vi "model torque calculation3MathScript.vi"() -> ()   [LabVIEW 2019]
uses:
  <vilib>/imath/engines/lvmath2/RunTimeEngine/NodeEndStatement/NIMS_NodeEndStatement_Output.vi
  <instcachedir>/0/NIMS_NodeEndStatement_Output_53EC0D466D134D7ABD903AC30B43404B.lvgen/NIMS_NodeEndStatement_Output_53EC0D466D134D7ABD903AC30B43404B_001.vi
  <vilib>/imath/engines/lvmath2/RunTimeEngine/ErrorHandling/NIMS_Finalize Error.vi
panel:
  out "lower leg(l2)":dbl(slide) scale=8.0..48.0
  out "foot(l3)":dbl(slide) scale=2.0..12.0
  out "thigh(l1)":dbl(slide) scale=8.0..48.0
  out "Tknee":dbl(slide) scale=-100.0..200.0
  out "Tankle":dbl(slide) scale=-100.0..200.0
  out "Thip":dbl(slide) scale=-100.0..200.0
  in  "?":dbl(slide) scale=40.0..190.0
  in  "Ankle_è3":dbl(slide) scale=-45.0..45.0
  in  "Knee_è2":dbl(slide) scale=0.0..145.0
  in  "hip_è1":dbl(slide) scale=-10.0..145.0
  in  "Select Model BSP":bool
  in  "Select sex":bool
  out "KneeD_m4":dbl(slide) scale=0.0..35.0
  out "FootD_m3":dbl(slide) scale=0.0..4.0
  out "LowerLegD_m2":dbl(slide) scale=0.0..10.0
  out "ThighD_m1":dbl(slide) scale=0.0..25.0 scale format="%#.8g"
  in  "?":dbl(slide) scale=20.0..170.0
  # "CALCULATION OF BASIC SIZES OF ROBOTIC EXTRACTUAL LOWER LIMB"
  # "KINEMATIC ANALYSIS"
  # "Á.Calculate the mass of each member of the lower limb in relation to its total mass"
  # "Mass Segment Body to Model Dempster BSP"
  # "Select Total Mass(Kg)"
  # "Zatsiorsky BSP"
  # "Dempster BSP"
  # "Males"
  # "Female"
  # "B.Calculation of moments of each segment  of the lower right extremity in relation to the total mass (kg) its height (m) and the change of angles of each joints."
  # "Select Angles"
  # "Select Height(h)"
  # "Length(cm)"
  # "Flexion/extension"
  # "m"
  # "Nm"
  # "Nm"
  # "Nm"
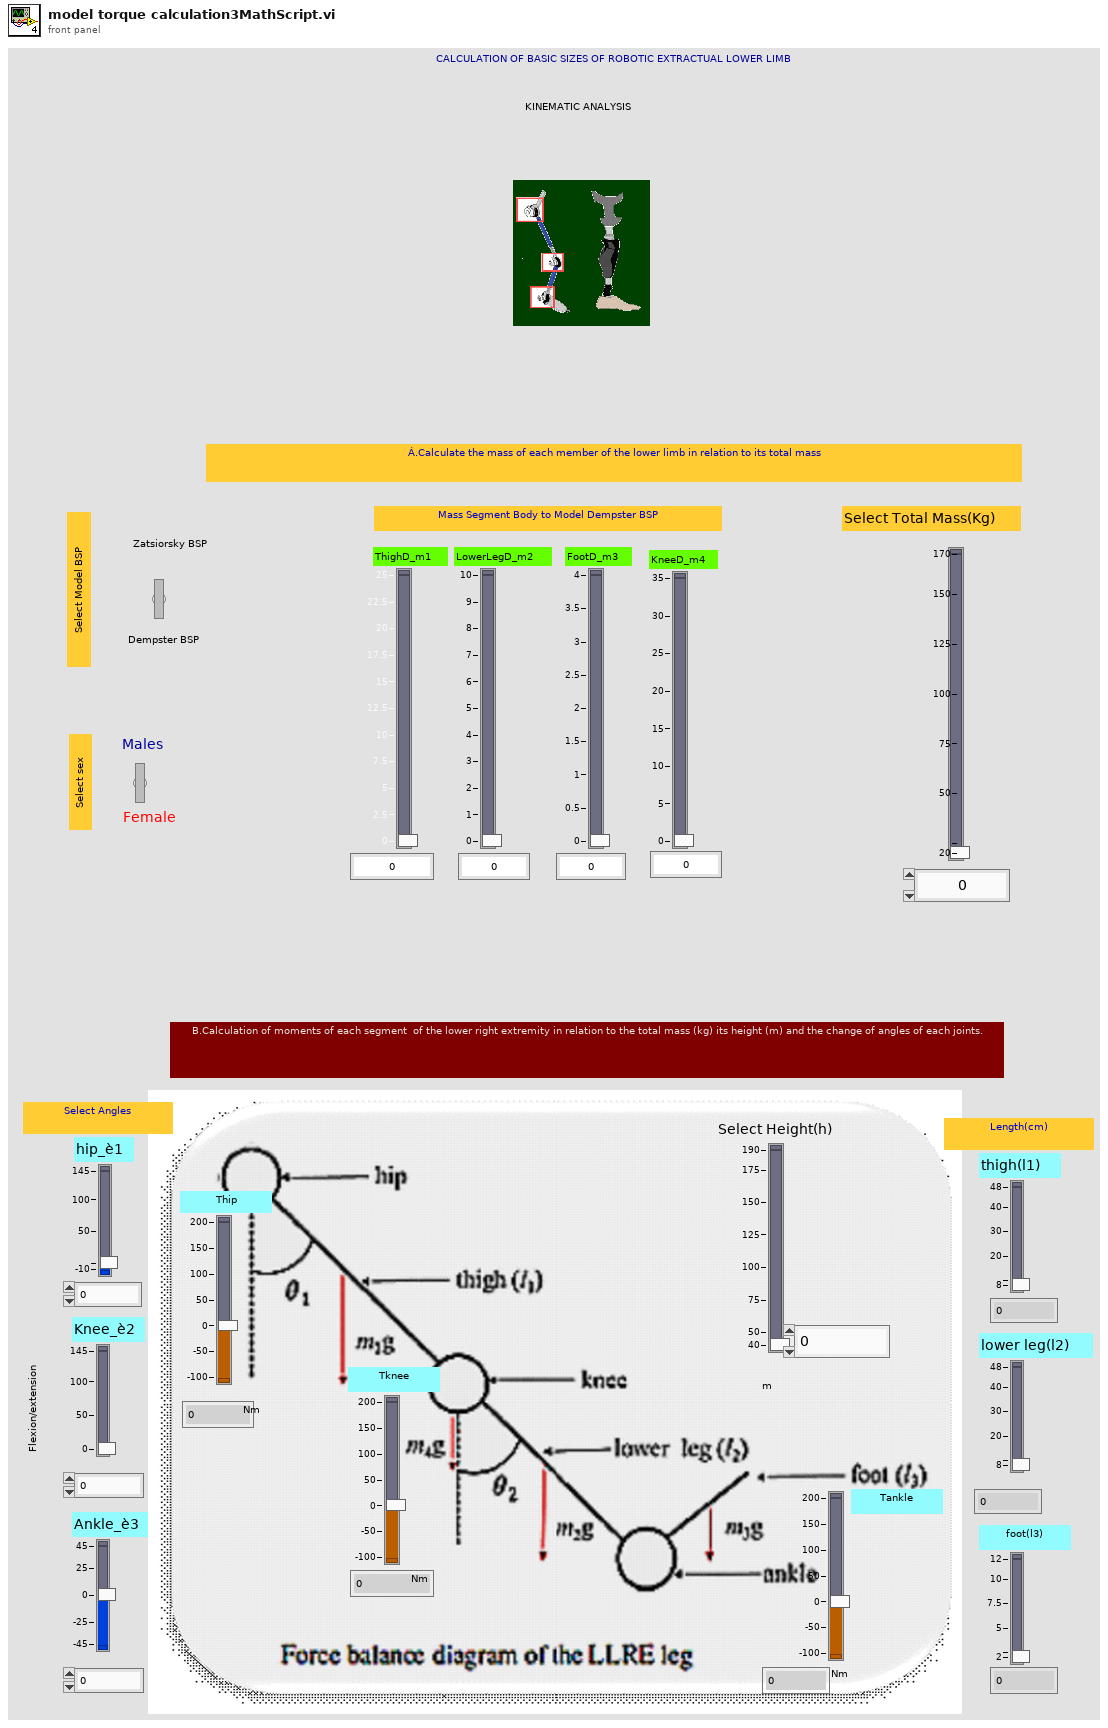
[diagram p1: front panel]
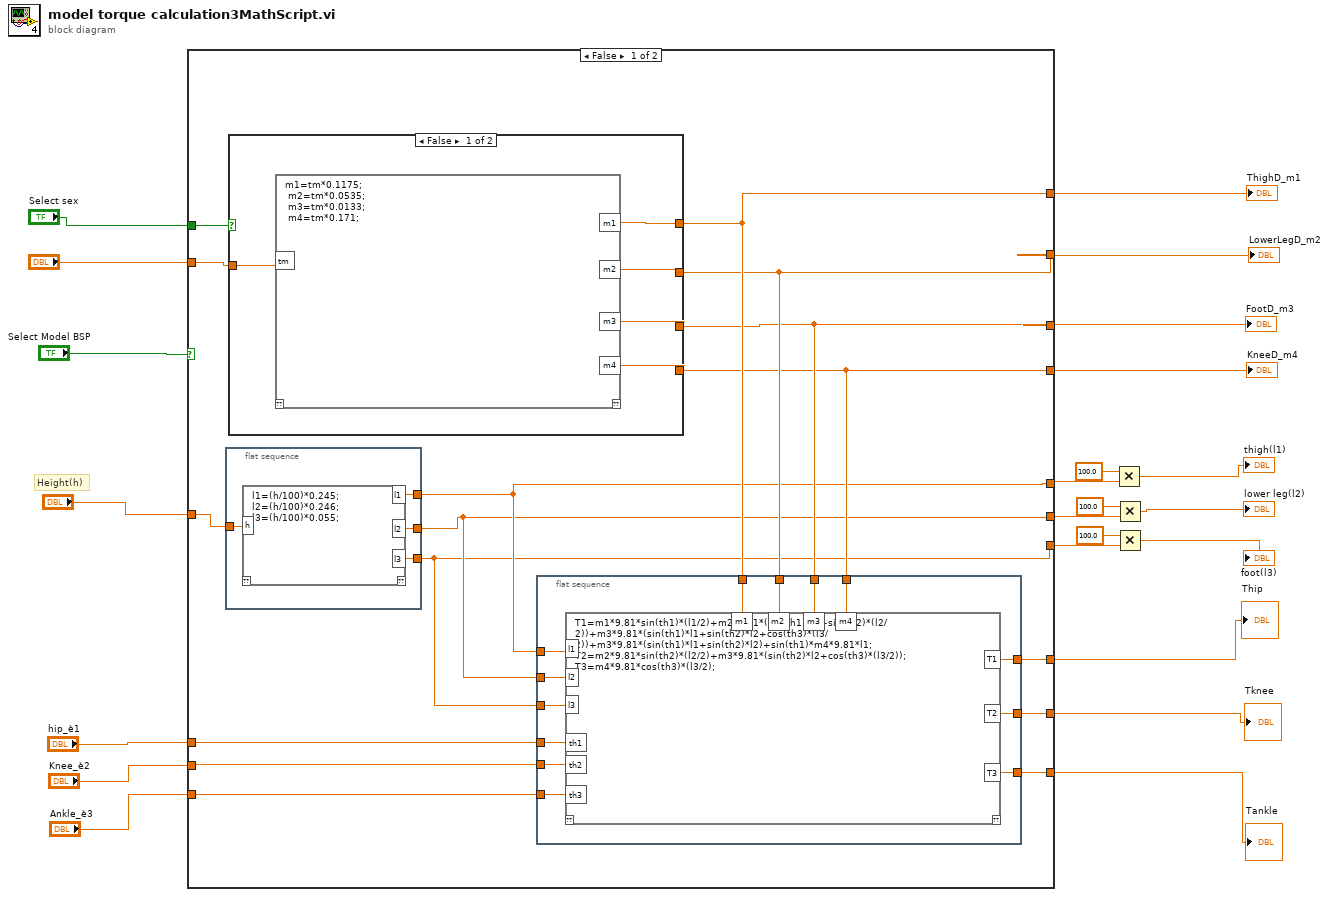
[diagram p0: block diagram]
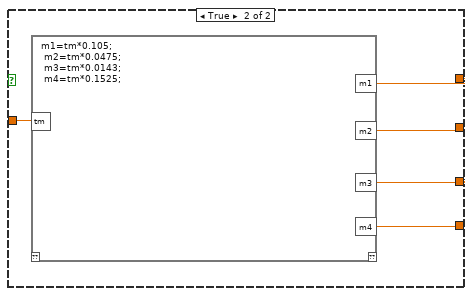
[diagram p2: hidden frame]
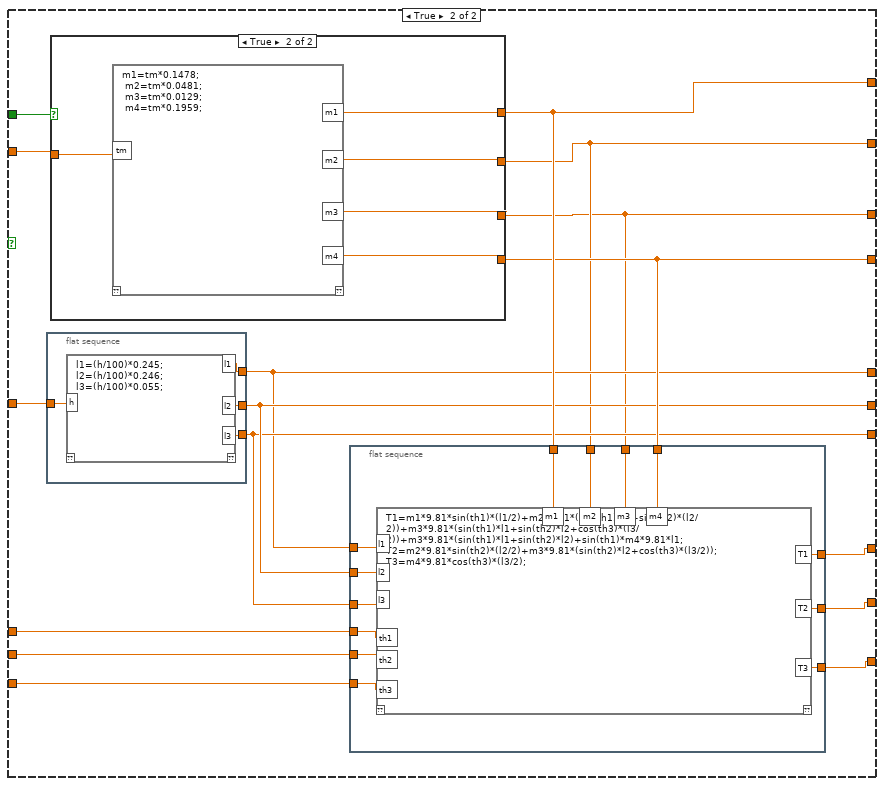
[diagram p3: hidden frame]
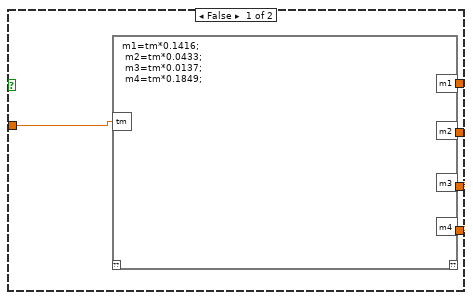
[diagram p4: hidden frame]
diagram:
  # "Height(h)"
  n1 = case shown="False" "Select Model BSP" {
    tunnel: "Select sex" -> [w39 w346]
    tunnel: "?" -> [w38 w345]
    tunnel: [w36 w340] -> w20
    tunnel: [w35 w332] -> w19
    tunnel: [w34 w331] -> w18
    tunnel: [w33 w339] -> w17
    tunnel: "?" -> [w37 w344]
    tunnel: "hip_è1" -> [w32 w343]
    tunnel: "Knee_è2" -> [w31 w342]
    tunnel: "Ankle_è3" -> [w30 w341]
    tunnel: [w29 w338] -> w12
    tunnel: [w28 w337] -> w11
    tunnel: [w27 w336] -> w10
    tunnel: [w25 w335] -> w4
    tunnel: [w24 w334] -> w2
    tunnel: [w26 w333] -> w9
    frame False {
      n2 = flat-sequence {
        tunnel: w37 -> [w191]
        tunnel: [w190] -> w26
        tunnel: [w189] -> w25
        tunnel: [w188] -> w24
        frame #0 {
          n3 = mathscript code="l1=(h/100)*0.245;\nl2=(h/100)*0.246;\nl3=(h/100)*0.055;"("h"=w191) -> ("l1"=w190:dbl, "l2"=w189:dbl, "l3"=w188:dbl)  [unwired: 1 in, 1 out]
        }
      }
      n4 = case shown="False" w39 {
        tunnel: [w235 w283] -> w33
        tunnel: [w236 w284] -> w34
        tunnel: [w237 w285] -> w35
        tunnel: w38 -> [w233 w286]
        tunnel: [w234 w282] -> w36
        frame False {
          n5 = mathscript code="m1=tm*0.1175;\n m2=tm*0.0535;\n m3=tm*0.0133;\n m4=tm*0.171;"("tm"=w233) -> ("m1"=w234:dbl, "m2"=w237:dbl, "m3"=w236:dbl, "m4"=w235:dbl)  [unwired: 1 in, 1 out]
        }
        frame True {
          n6 = mathscript code="m1=tm*0.105;\n m2=tm*0.0475;\n m3=tm*0.0143;\n m4=tm*0.1525;"("tm"=w286) -> ("m1"=w282:dbl, "m2"=w285:dbl, "m3"=w284:dbl, "m4"=w283:dbl)  [unwired: 1 in, 1 out]
        }
      }
      n7 = flat-sequence {
        tunnel: w36 -> [w52]
        tunnel: w35 -> [w51]
        tunnel: w34 -> [w50]
        tunnel: w33 -> [w49]
        tunnel: w32 -> [w48]
        tunnel: w31 -> [w47]
        tunnel: w30 -> [w46]
        tunnel: [w45] -> w29
        tunnel: [w44] -> w28
        tunnel: [w43] -> w27
        tunnel: w26 -> [w42]
        tunnel: w25 -> [w41]
        tunnel: w24 -> [w40]
        frame #0 {
          n8 = mathscript code="T1=m1*9.81*sin(th1)*(l1/2)+m2*9.81*(sin(th1)*l1+sin(th2)*(l2/2))+m3*9.81*(sin(th1)*l1+sin(th2)*l2+cos(th3)*(l3/2))+m3*9.81*(sin(th1)*l1+sin(th2)*l2)+sin(th1)*m4*9.81*l1;\nT2=m2*9.81*sin(th2)*(l2/2)+m3*9.81*(sin(th2)*l2+cos(th3)*(l3/2));\nT3=m4*9.81*cos(th3)*(l3/2);"("m1"=w52, "m2"=w51, "m3"=w50, "m4"=w49, "l1"=w42, "l2"=w41, "l3"=w40, "th1"=w48, "th2"=w47, "th3"=w46) -> ("T1"=w45:dbl, "T2"=w44:dbl, "T3"=w43:dbl)  [unwired: 1 in, 1 out]
        }
      }
    }
    frame True {
      n9 = flat-sequence {
        tunnel: w344 -> [w498]
        tunnel: [w497] -> w335
        tunnel: [w496] -> w334
        tunnel: [w495] -> w333
        frame #0 {
          n10 = mathscript code="l1=(h/100)*0.245;\nl2=(h/100)*0.246;\nl3=(h/100)*0.055;"("h"=w498) -> ("l1"=w495:dbl, "l2"=w497:dbl, "l3"=w496:dbl)  [unwired: 1 in, 1 out]
        }
      }
      n11 = case shown="True" w346 {
        tunnel: [w542 w590] -> w339
        tunnel: [w543 w591] -> w331
        tunnel: [w544 w592] -> w332
        tunnel: w345 -> [w540 w593]
        tunnel: [w541 w589] -> w340
        frame False {
          n12 = mathscript code="m1=tm*0.1416;\n m2=tm*0.0433;\n m3=tm*0.0137;\n m4=tm*0.1849;"("tm"=w540) -> ("m1"=w541:dbl, "m2"=w544:dbl, "m3"=w543:dbl, "m4"=w542:dbl)  [unwired: 1 in, 1 out]
        }
        frame True {
          n13 = mathscript code="m1=tm*0.1478;\n m2=tm*0.0481;\n m3=tm*0.0129;\n m4=tm*0.1959;"("tm"=w593) -> ("m1"=w589:dbl, "m2"=w592:dbl, "m3"=w591:dbl, "m4"=w590:dbl)  [unwired: 1 in, 1 out]
        }
      }
      n14 = flat-sequence {
        tunnel: w343 -> [w359]
        tunnel: w342 -> [w358]
        tunnel: w341 -> [w357]
        tunnel: w340 -> [w356]
        tunnel: w339 -> [w355]
        tunnel: [w354] -> w338
        tunnel: [w353] -> w337
        tunnel: [w352] -> w336
        tunnel: w335 -> [w351]
        tunnel: w334 -> [w350]
        tunnel: w333 -> [w349]
        tunnel: w332 -> [w348]
        tunnel: w331 -> [w347]
        frame #0 {
          n15 = mathscript code="T1=m1*9.81*sin(th1)*(l1/2)+m2*9.81*(sin(th1)*l1+sin(th2)*(l2/2))+m3*9.81*(sin(th1)*l1+sin(th2)*l2+cos(th3)*(l3/2))+m3*9.81*(sin(th1)*l1+sin(th2)*l2)+sin(th1)*m4*9.81*l1;\nT2=m2*9.81*sin(th2)*(l2/2)+m3*9.81*(sin(th2)*l2+cos(th3)*(l3/2));\nT3=m4*9.81*cos(th3)*(l3/2);"("m1"=w356, "m2"=w348, "m3"=w347, "m4"=w355, "l1"=w349, "l2"=w351, "l3"=w350, "th1"=w359, "th2"=w358, "th3"=w357) -> ("T1"=w354:dbl, "T2"=w353:dbl, "T3"=w352:dbl)  [unwired: 1 in, 1 out]
        }
      }
    }
  }
  "ThighD_m1" <- w20
  "LowerLegD_m2" <- w19
  "FootD_m3" <- w18
  "KneeD_m4" <- w17
  "Thip" <- w12
  "Tknee" <- w11
  "Tankle" <- w10
  n16 = Multiply(x=100.0, y=w9) -> (x*y=→"thigh(l1)":dbl)
  n17 = Multiply(x=100.0, y=w4) -> (x*y=→"lower leg(l2)":dbl)
  n18 = Multiply(x=100.0, y=w2) -> (x*y=→"foot(l3)":dbl)
